vi "Select Function Type.vi"(8 "error in (no error)":errorcluster, 10 "Function Type":T1, 11 "PXIe5413 in":refnum<class "PXIe5413.lvclass">) -> (0 "error out":errorcluster, 3 "PXIe5413 out":refnum<class "PXIe5413.lvclass">)   [LabVIEW 2018, in "PXIe5413.lvlib" / "PXIe5413.lvclass"]
uses:
  PXIe5413.lvclass
  PPLs/Function Generator/Parent/Function Generator.lvlibp/Custom Controls/Function Type.ctl
  <instrlib>/niFgen/niFgen.llb/niFgen Output Mode.ctl
  PPLs/Function Generator/Parent/Function Generator.lvlibp/Function Generator.lvclass
  C:/Projects/LabVIEW/PPLs/Function Generator/Parent/Function Generator.lvlibp/Function Generator.lvclass
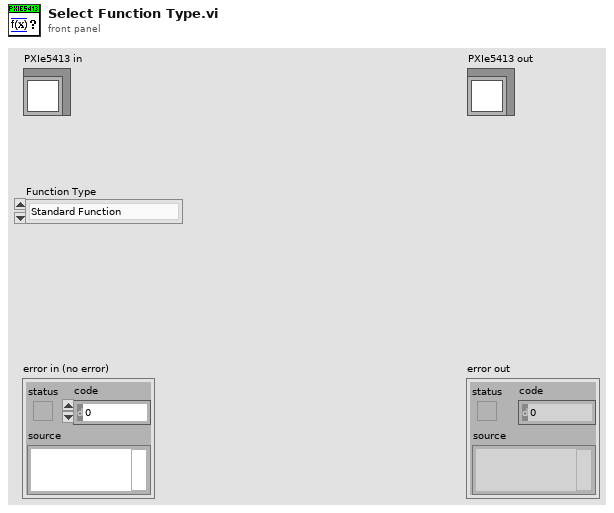
[diagram p1: front panel]
types:
  T1 = typedef "Function Generator.lvlibp/Function Generator.lvclass/Function Type.ctl" = enum16{"Standard Function", "Arbitrary Waveform", "Frequency List", "Arbitrary Sequence", "Script"}
  T2 = typedef "niFgen Output Mode.ctl" = u32
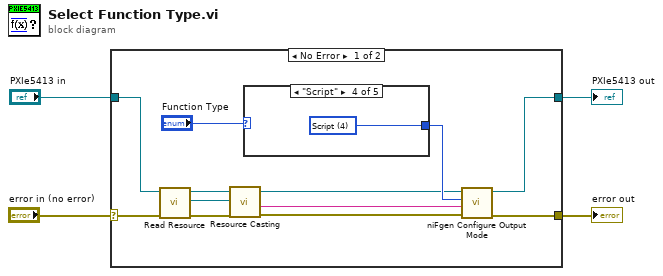
[diagram p0: block diagram]
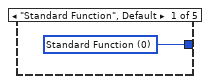
[diagram p2: hidden frame]
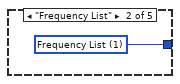
[diagram p3: hidden frame]
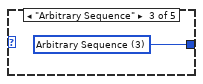
[diagram p4: hidden frame]
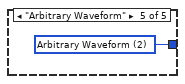
[diagram p5: hidden frame]
diagram:
  n1 = case shown="No Error" "error in (no error)" {
    selector: "error in (no error)" -> [w15 w22]
    tunnel: [w6 w22] -> w3
    tunnel: [w7 w21] -> w2
    tunnel: "PXIe5413 in" -> [w14 w21]
    frame No Error {
      n2 = call "Read Resource.vi"("error in (no error)"=w15, "Function Generator in"=w14) -> ("error out"=w13:errorcluster, "Resource"=w5:refnum<visa-resource-name>, "Function Generator out"=w9:refnum<class "PXIe5413.lvclass">)  [unwired: 7 in]
      n3 = call "Resource Casting.vi"("error in (no error)"=w13, "VISA Resource In"=w5, "PXIe5413 in"=w9) -> ("error out"=w11:errorcluster, "Casted Resource"=w12:string, "PXIe5413 out"=w7:refnum<class "PXIe5413.lvclass">)  [unwired: 6 in]
      n4 = case shown="\"Script\"" "Function Type" {
        tunnel: [w16 w17 w18 w19 w20] -> w10
        frame "Standard Function", Default {
          w16 = T2 0 items=["Standard Function", "Frequency List", "Arbitrary Waveform", "Arbitrary Sequence", "Script"] ("Output Mode (default: 0=Standard Function)")
        }
        frame "Frequency List" {
          w17 = T2 1 items=["Standard Function", "Frequency List", "Arbitrary Waveform", "Arbitrary Sequence", "Script"] ("Output Mode (default: 0=Standard Function)")
        }
        frame "Arbitrary Sequence" {
          w18 = T2 3 items=["Standard Function", "Frequency List", "Arbitrary Waveform", "Arbitrary Sequence", "Script"] ("Output Mode (default: 0=Standard Function)")
        }
        frame "Script" {
          w19 = T2 4 items=["Standard Function", "Frequency List", "Arbitrary Waveform", "Arbitrary Sequence", "Script"] ("Output Mode (default: 0=Standard Function)")
        }
        frame "Arbitrary Waveform" {
          w20 = T2 2 items=["Standard Function", "Frequency List", "Arbitrary Waveform", "Arbitrary Sequence", "Script"] ("Output Mode (default: 0=Standard Function)")
        }
      }
      n5 = call <instrlib>:"niFgen Configure Output Mode.vi"("error in (no error)"=w11, "Output Mode (default: 0=Standard Function)"=w10, "Instrument Handle"=w12) -> ("error out"=w6:errorcluster)  [unwired: 6 in, 1 out]
    }
    frame Error {
    }
  }
  "error out" <- w3
  "PXIe5413 out" <- w2
